vi "SDLEDUPDT.vi"(8 "error in (no error)":errorcluster, 10 "Command":string, 11 "UI Actor in":refnum<class "UI Actor.lvclass">) -> (0 "error out":errorcluster)   [LabVIEW 2020, in "UI Actor.lvlib" / "UI Actor.lvclass"]
uses:
  UI Actor.lvclass
  UI Actor.lvclass/UI Actor.ctl
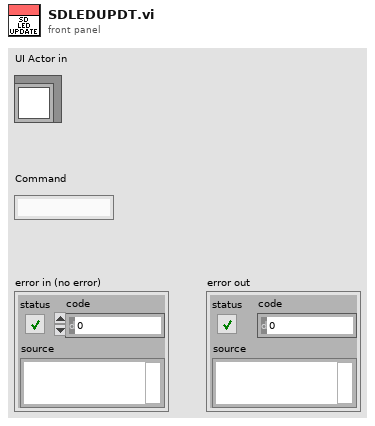
[diagram p1: front panel]
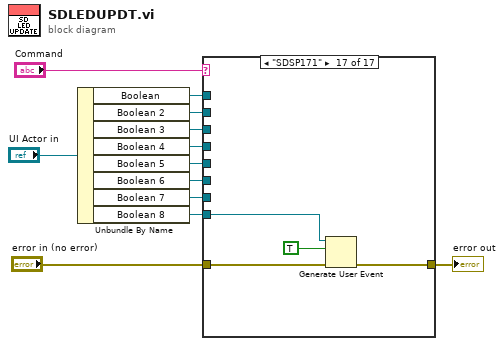
[diagram p0: block diagram]
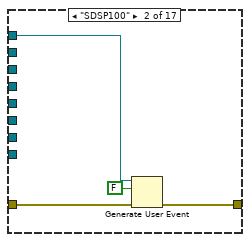
[diagram p3: hidden frame]
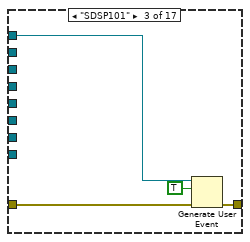
[diagram p4: hidden frame]
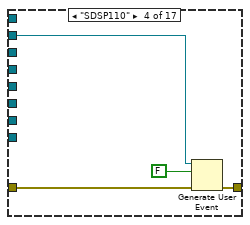
[diagram p5: hidden frame]
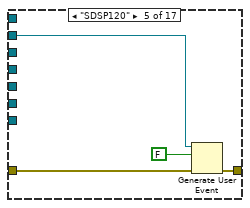
[diagram p6: hidden frame]
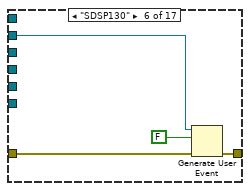
[diagram p7: hidden frame]
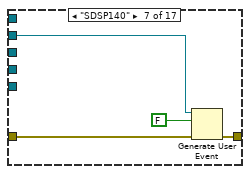
[diagram p8: hidden frame]
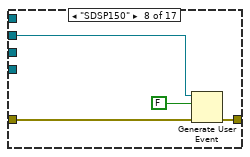
[diagram p9: hidden frame]
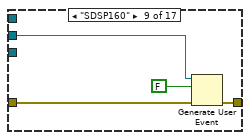
[diagram p10: hidden frame]
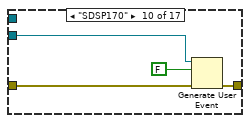
[diagram p11: hidden frame]
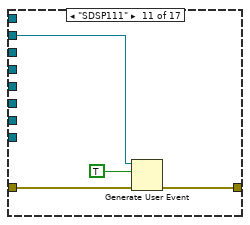
[diagram p12: hidden frame]
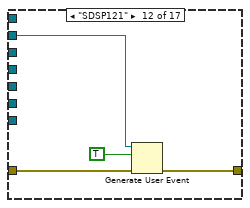
[diagram p13: hidden frame]
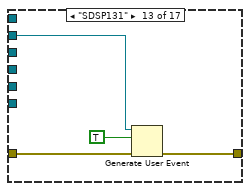
[diagram p14: hidden frame]
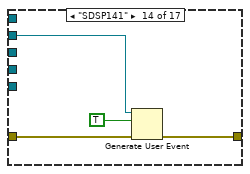
[diagram p15: hidden frame]
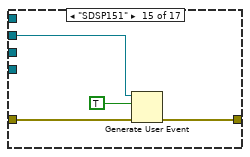
[diagram p16: hidden frame]
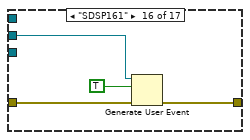
[diagram p17: hidden frame]
diagram:
  n1 = Unbundle By Name("UI Actor in") -> ("Boolean"=w5:refnum<user-event>, "Boolean 2"=w6:refnum<user-event>, "Boolean 3"=w7:refnum<user-event>, "Boolean 4"=w8:refnum<user-event>, "Boolean 5"=w9:refnum<user-event>, "Boolean 6"=w10:refnum<user-event>, "Boolean 7"=w11:refnum<user-event>, "Boolean 8"=w1:refnum<user-event>)
  n2 = case shown="\"SDSP171\"" "Command" {
    tunnel: w1 -> [_ _ _ _ _ _ _ _ _ w45 _ _ _ _ _ _ w73]
    tunnel: "error in (no error)" -> [_ w16 w20 w24 w28 w32 w36 w40 w44 w48 w52 w56 w60 w64 w68 w72 w76]
    tunnel: [_ w15 w19 w23 w27 w31 w35 w39 w43 w47 w51 w55 w59 w63 w67 w71 w75] -> w3
    tunnel: w5 -> [_ w14 w18 _ _ _ _ _ _ _ _ _ _ _ _ _ _]
    tunnel: w6 -> [_ _ _ w22 _ _ _ _ _ _ w50 _ _ _ _ _ _]
    tunnel: w7 -> [_ _ _ _ w25 _ _ _ _ _ _ w53 _ _ _ _ _]
    tunnel: w8 -> [_ _ _ _ _ w29 _ _ _ _ _ _ w57 _ _ _ _]
    tunnel: w9 -> [_ _ _ _ _ _ w33 _ _ _ _ _ _ w61 _ _ _]
    tunnel: w10 -> [_ _ _ _ _ _ _ w37 _ _ _ _ _ _ w65 _ _]
    tunnel: w11 -> [_ _ _ _ _ _ _ _ w41 _ _ _ _ _ _ w69 _]
    frame "False", Default {
    }
    frame "SDSP100" {
      n3 = Generate User Event(user event=w14, event data cluster=FALSE ("event data"), error in=w16) -> (error out=w15:errorcluster)  [unwired: 1 in, 1 out]
    }
    frame "SDSP101" {
      n4 = Generate User Event(user event=w18, event data cluster=TRUE ("event data"), error in=w20) -> (error out=w19:errorcluster)  [unwired: 1 in, 1 out]
    }
    frame "SDSP110" {
      n5 = Generate User Event(user event=w22, event data cluster=FALSE ("event data"), error in=w24) -> (error out=w23:errorcluster)  [unwired: 1 in, 1 out]
    }
    frame "SDSP120" {
      n6 = Generate User Event(user event=w25, event data cluster=FALSE ("event data"), error in=w28) -> (error out=w27:errorcluster)  [unwired: 1 in, 1 out]
    }
    frame "SDSP130" {
      n7 = Generate User Event(user event=w29, event data cluster=FALSE ("event data"), error in=w32) -> (error out=w31:errorcluster)  [unwired: 1 in, 1 out]
    }
    frame "SDSP140" {
      n8 = Generate User Event(user event=w33, event data cluster=FALSE ("event data"), error in=w36) -> (error out=w35:errorcluster)  [unwired: 1 in, 1 out]
    }
    frame "SDSP150" {
      n9 = Generate User Event(user event=w37, event data cluster=FALSE ("event data"), error in=w40) -> (error out=w39:errorcluster)  [unwired: 1 in, 1 out]
    }
    frame "SDSP160" {
      n10 = Generate User Event(user event=w41, event data cluster=FALSE ("event data"), error in=w44) -> (error out=w43:errorcluster)  [unwired: 1 in, 1 out]
    }
    frame "SDSP170" {
      n11 = Generate User Event(user event=w45, event data cluster=FALSE ("event data"), error in=w48) -> (error out=w47:errorcluster)  [unwired: 1 in, 1 out]
    }
    frame "SDSP111" {
      n12 = Generate User Event(user event=w50, event data cluster=TRUE ("event data"), error in=w52) -> (error out=w51:errorcluster)  [unwired: 1 in, 1 out]
    }
    frame "SDSP121" {
      n13 = Generate User Event(user event=w53, event data cluster=TRUE ("event data"), error in=w56) -> (error out=w55:errorcluster)  [unwired: 1 in, 1 out]
    }
    frame "SDSP131" {
      n14 = Generate User Event(user event=w57, event data cluster=TRUE ("event data"), error in=w60) -> (error out=w59:errorcluster)  [unwired: 1 in, 1 out]
    }
    frame "SDSP141" {
      n15 = Generate User Event(user event=w61, event data cluster=TRUE ("event data"), error in=w64) -> (error out=w63:errorcluster)  [unwired: 1 in, 1 out]
    }
    frame "SDSP151" {
      n16 = Generate User Event(user event=w65, event data cluster=TRUE ("event data"), error in=w68) -> (error out=w67:errorcluster)  [unwired: 1 in, 1 out]
    }
    frame "SDSP161" {
      n17 = Generate User Event(user event=w69, event data cluster=TRUE ("event data"), error in=w72) -> (error out=w71:errorcluster)  [unwired: 1 in, 1 out]
    }
    frame "SDSP171" {
      n18 = Generate User Event(user event=w73, event data cluster=TRUE ("event data"), error in=w76) -> (error out=w75:errorcluster)  [unwired: 1 in, 1 out]
    }
  }
  "error out" <- w3
